vi "Change Behavior.vi"(8 "error in":errorcluster, 10 "New Behavior":refnum<class "Flex UI.lvclass">, 11 "Philips UI in":refnum<class "Flex UI.lvclass">) -> (0 "error out":errorcluster, 3 "Philips UI out":refnum<class "Flex UI.lvclass">)   [LabVIEW 2014, in "Flex UI.lvclass"]
uses:
  Flex UI.lvclass
  Flex UI.lvclass/Flex UI.ctl
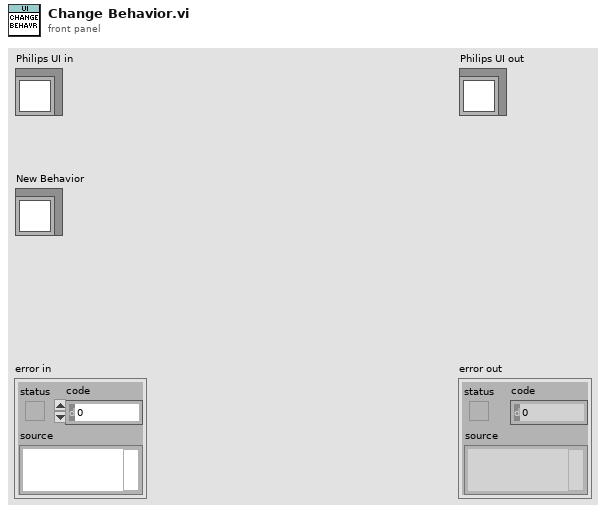
[diagram p1: front panel]
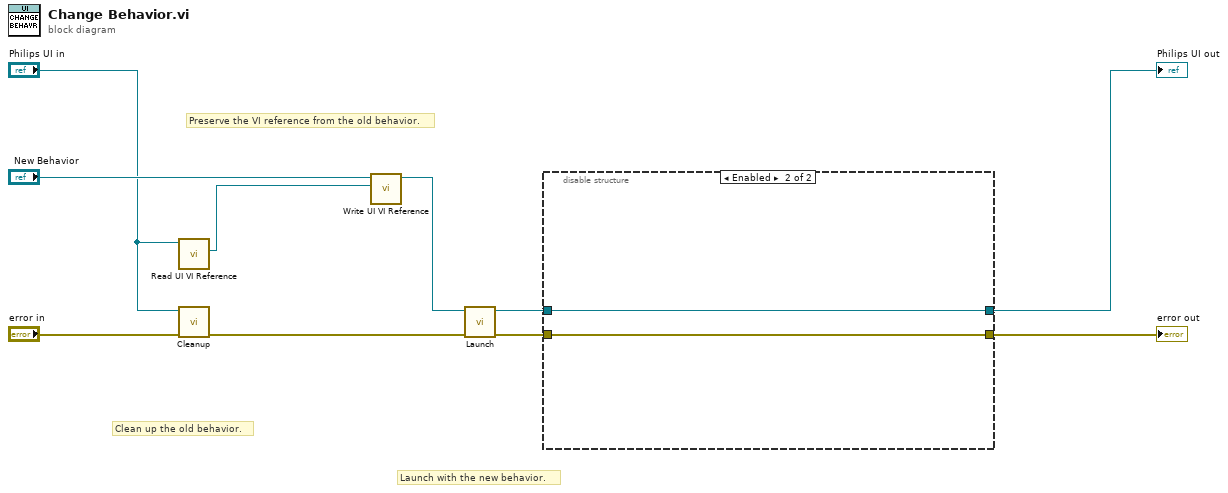
[diagram p0: block diagram]
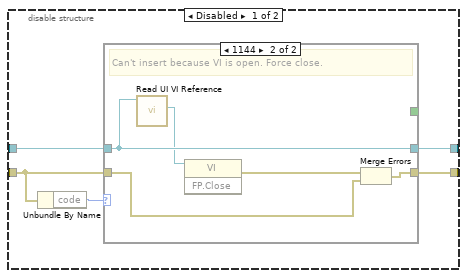
[diagram p2: hidden frame]
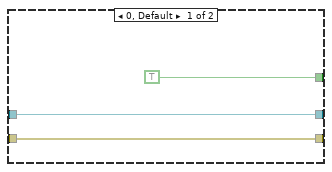
[diagram p3: hidden frame]
diagram:
  # "Preserve the VI reference from the old behavior."
  # "Launch with the new behavior."
  # "Clean up the old behavior."
  n1 = call "Read UI VI Reference.vi"("Philips UI in"="Philips UI in") -> ("UI VI Reference"=w6:refnum<vi>)  [unwired: 9 in, 1 out]
  n2 = call-dynamic "Cleanup.vi"("error in"="error in", "Philips UI in"="Philips UI in") -> ("error out"=w9:errorcluster)  [unwired: 9 in]
  n3 = call "Write UI VI Reference.vi"("UI VI Reference"=w6, "Philips UI in"="New Behavior") -> ("Philips UI out"=w4:refnum<class "Flex UI.lvclass">)  [unwired: 9 in]
  n4 = call-dynamic "Launch.vi"("error in"=w9, "Philips UI in"=w4) -> ("error out"=w1:errorcluster, "Philips UI out"=w2:refnum<class "Flex UI.lvclass">)  [unwired: 8 in]
  n5 = disable-structure shown="Enabled" {
    disable-tunnel: [w15 w24] -> w5
    disable-tunnel: [w14 w25] -> w3
    disable-tunnel: w2 -> [w12 w25]
    disable-tunnel: w1 -> [w11 w24]
    frame Disabled {
      n6 = Unbundle By Name(w11) -> ("code"=w13:i32)
      n7 = case shown="1144" w13 {
        tunnel: [w18 w23] -> w14
        tunnel: w12 -> [w18 w23]
        tunnel: [w17 w20] -> w15
        tunnel: w11 -> [w17 w19]
        tunnel: [TRUE _] -> _
        frame 0, Default {
        }
        frame 1144 {
          # "Can't insert because VI is open. Force close."
          n8 = call "Read UI VI Reference.vi"("Philips UI in"=w23) -> ("UI VI Reference"=w21:refnum<vi>)  [unwired: 9 in, 1 out]
          n9 = invoke class="VI" method="FP.Close"(reference=w21) -> (error out=w22:errorcluster)  [unwired: 2 in, 2 out]
          n10 = Merge Errors(w22, w19) -> (w20:errorcluster)
        }
      }
    }
    frame Enabled {
    }
  }
  "error out" <- w5
  "Philips UI out" <- w3
